vi "Main.vi"() -> ()   [LabVIEW 2019]
uses:
  <vilib>/sound2/lvsound2.llb/Sound Data Format.ctl
  <vilib>/sound2/lvsound2.llb/Sampling Mode.ctl
  647fc178-2e3b-49ce-a191-7d700641073f.vi
  <vilib>/sound2/lvsound2.llb/Sound Input Read (DBL).vi
  <vilib>/measure/macond.llb/IIR Filter for N Chan.vi
  <vilib>/measure/maspectr.llb/FFT Power Spectrum and PSD for N Chan.vi
  <vilib>/measure/NI_MAPro.lvlib
panel:
  out "Spectrum Data":cluster{"f0":dbl, "df":dbl, "magnitude":dbl[]}[](graph)
  out "Raw Data":waveform(dbl)[](graph)
  out "error out":errorcluster
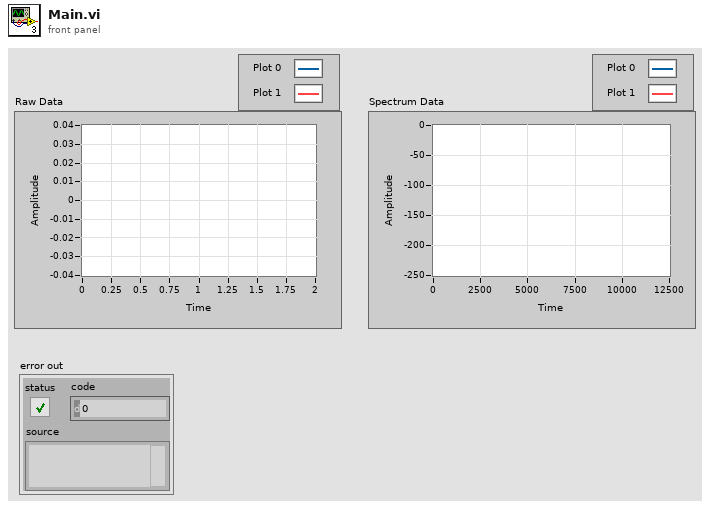
[diagram p1: front panel]
types:
  T1 = cluster{"Topology":enum16{"Off", "Butterworth", "Chebyshev", "Inverse Chebyshev", "Elliptic", "Bessel"}, "Type":enum16{"Lowpass", "Highpass", "Bandpass", "Bandstop"}, "Order":i32, "Lower Fc":dbl, "Upper Fc":dbl, "PB Ripple":dbl, "SB Attenuation":dbl}
  T2 = typedef "Sampling Mode.ctl" = i32
  T3 = typedef "Sound Data Format.ctl" = cluster{"sample rate (S/s)":dbl, "number of channels":i32, "bits per sample":i32}
  T4 = typedef "Sound Input Task ID.ctl" = u32
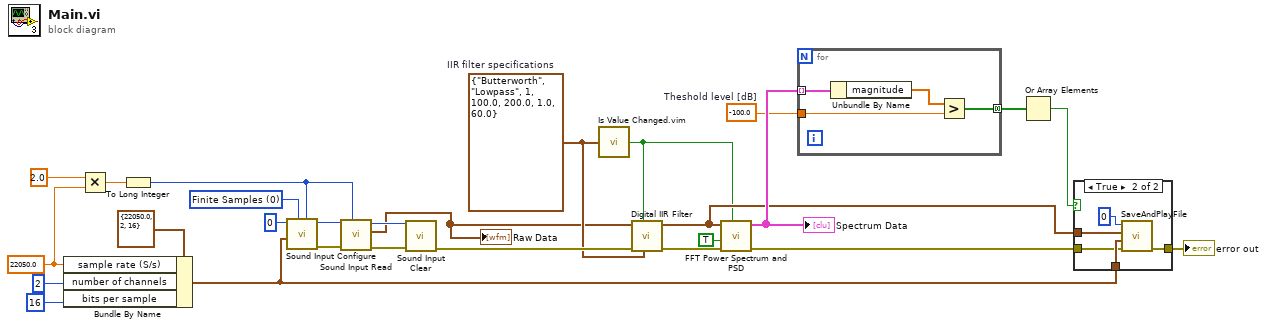
[diagram p0: block diagram]
diagram:
  w3 = -100.0  # Theshold level [dB]
  w10 = T1 {"Topology"=enum."Butterworth", "Type"=enum."Lowpass", "Order"=1, "Lower Fc"=100.0, "Upper Fc"=200.0, "PB Ripple"=1.0, "SB Attenuation"=60.0}  # IIR filter specifications
  w20 = T2 0 items=["Finite Samples", "Continuous Samples"] ("sample mode")
  w14 = 22050.0 ("Sample rate (Hz)")
  n1 = Bundle By Name(cluster=T3 {"sample rate (S/s)"=22050.0, "number of channels"=2, "bits per sample"=16} ("Sound Format"), "sample rate (S/s)"=w14, "number of channels"=2 ("#Channels"), "bits per sample"=16 ("Resolution (bits)")) -> (w13:T3)
  n2 = Multiply(x=2.0 ("Duration (s)"), y=w14) -> (x*y=w18:dbl)
  n3 = To Long Integer(number=w18) -> (32bit integer=w17:i32)
  n4 = call <vilib>:"Sound Input Configure.vi"("number of samples/ch"=w17, "sample mode"=w20, "sound format"=w13, "device ID"=u32 0 ("Device")) -> ("error out"=w23:errorcluster, "task ID"=w19:T4)  [unwired: 6 in]
  n5 = call-poly <vilib>:"Sound Input Read.vi"("number of samples/ch"=w17, "error in (no error)"=w23, "task ID"=w19) -> ("error out"=w15:errorcluster, "data"=w7:waveform(dbl)[], "task ID out"=w16:T4)  [unwired: 6 in]
  "Raw Data" <- w7
  n6 = call <vilib>:"Sound Input Clear.vi"("error in (no error)"=w15, "task ID"=w16) -> ("error out"=w12:errorcluster)  [unwired: 9 in]
  n7 = call "Is Value Changed.vim"("value"=w10) -> ("changed or first call?"=w5:bool)
  n8 = call-poly <vilib>:"Digital IIR Filter.vi"("IIR filter specifications"=w10, "reset filters"=w5, "error in (no error)"=w12, "signal(s) in"=w7) -> ("error out"=w6:errorcluster, "signal(s) out"=w8:waveform(dbl)[])  [unwired: 5 in, 1 out]
  n9 = call-poly <vilib>:"FFT Power Spectrum and PSD.vi"("restart averaging (F)"=w5, "error in (no error)"=w6, "dB On (F)"=TRUE, "time signals"=w8) -> ("error out"=w11:errorcluster, "Power Spectrum / PSD"=w9:cluster{"f0":dbl, "df":dbl, "magnitude":dbl[]}[])  [unwired: 4 in, 2 out]
  "Spectrum Data" <- w9
  n10 = for {
    tunnel: [w30] -> w2 mode=concatenating
    tunnel: w9 -> [w29] mode=indexing
    tunnel: w3 -> [w28]
    n11 = Unbundle By Name(w29) -> ("magnitude"=w31:dbl[])
    n12 = Greater?(x=w31, y=w28) -> (0:w30:bool[])
  }
  n13 = Or Array Elements(Boolean array=w2) -> (logical OR=w1:bool)
  n14 = case shown="True" w1 {
    tunnel: [w32 w36] -> w24
    tunnel: w13 -> [_ w35]
    tunnel: w11 -> [w32 w34]
    tunnel: w8 -> [_ w33]
    frame False {
    }
    frame True {
      n15 = call "SaveAndPlayFile.vi"("error in (no error)"=w34, "Sound Format"=w35, "Waveform(s) in"=w33, "Speaker device ID"=u32 0 ("Device")) -> ("error out"=w36:errorcluster)  [unwired: 7 in]
    }
  }
  "error out" <- w24
